vi "hardwareconfig.vi"(1 "Channel Select":i32[](listbox)) -> (2 "Alll DAQmx Device Names":tag[](array[tag]))   [LabVIEW 2011]
panel:
  out "Array":void[](array[numeric])
  in  "GO":bool
  in  "Rescan":bool
  in  "Abort":bool
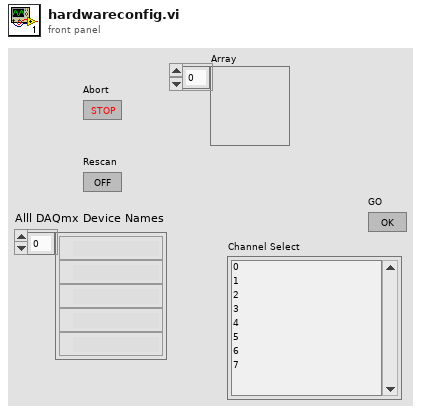
[diagram p1: front panel]
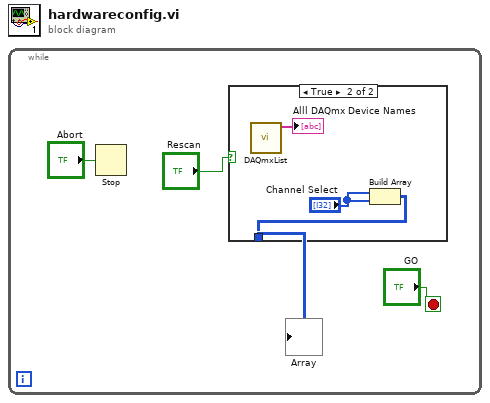
[diagram p0: block diagram]
diagram:
  n1 = while {
    stop <- "GO" stop-if-true
    n2 = Stop(stop? (T)="Abort") -> ()
    n3 = case shown="True" "Rescan" {
      tunnel: [_ w5] -> w1
      frame False {
      }
      frame True {
        n4 = call "DAQmxList.vi"() -> ("Alll DAQmx Device Names"=→"Alll DAQmx Device Names":tag[])  [unwired: 1 in, 3 out]
        n5 = Build Array("Channel Select", "Channel Select") -> (w5:i32[][])
      }
    }
    "Array" <- w1
  }
